vi "Add Application Search Path.vi"(8 "error in":errorcluster, 10 "New Search Path":path) -> (0 "error out":errorcluster, 1 "Added?":bool, 2 "Updated Search Paths":path[](array[path]), 5 "Initial Search Paths":path[](array[path]))   [LabVIEW 2020, in "VI-Hacker.lvlib"]
uses:
  VI-Hacker.lvlib
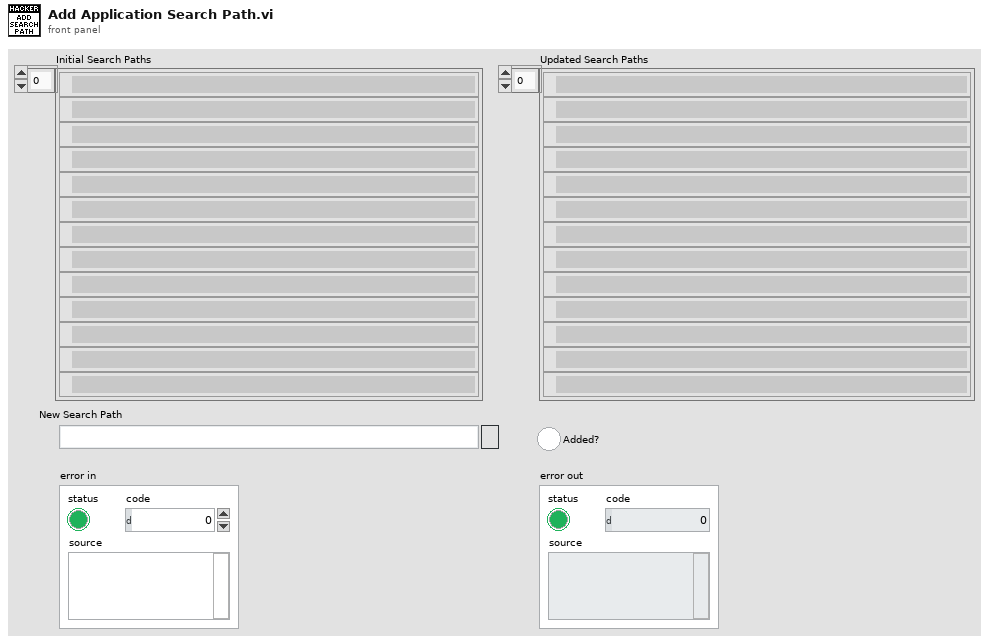
[diagram p1: front panel]
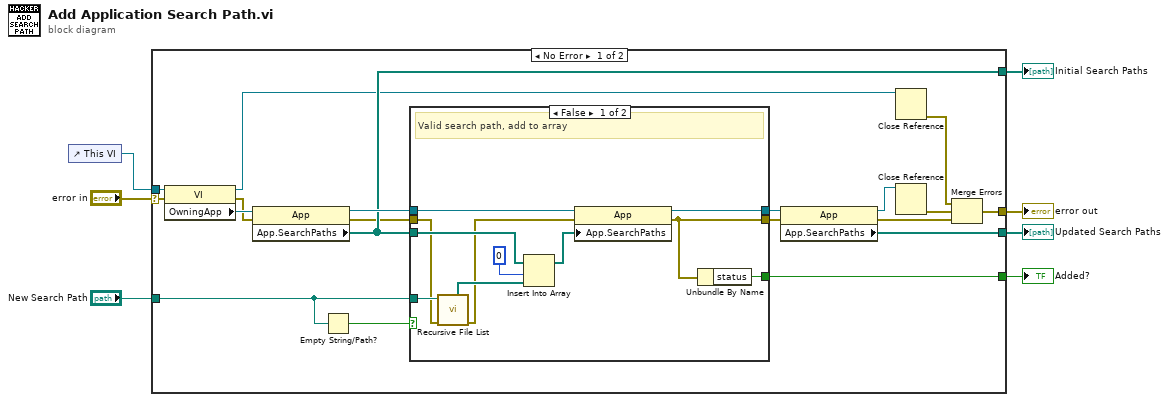
[diagram p0: block diagram]
diagram:
  n1 = control-ref of="This VI"() -> (w7:refnum<vi>)
  n2 = case shown="No Error" "error in" {
    selector: "error in" -> [w19 w40]
    tunnel: w7 -> [w26 _]
    tunnel: [w22 _] -> w6
    tunnel: [w21 _] -> w5
    tunnel: "New Search Path" -> [w8 _]
    tunnel: [w13 w40] -> w2
    tunnel: [w9 _] -> w1
    frame No Error {
      n3 = property class="VI"(reference=w26, error in=w19) -> (reference out=w14:refnum<vi>, error out=w15:errorcluster, "OwningApp"=w25:refnum<vi>)
      n4 = property class="App"(reference=w25, error in=w15) -> (reference out=w24:refnum<vi>, error out=w20:errorcluster, "App.SearchPaths"=w21:path[])
      n5 = Empty String/Path?(string/path=w8) -> (empty?=w10:bool)
      n6 = case shown="False" w10 {
        tunnel: w24 -> [w36 w38]
        tunnel: [w35 w38] -> w23
        tunnel: w21 -> [w34 _]
        tunnel: w20 -> [w28 w39]
        tunnel: w8 -> [w30 _]
        tunnel: [w32 w39] -> w18
        tunnel: [w31 _] -> w9
        frame False {
          # "Valid search path, add to array"
          n7 = call <vilib>:"Recursive File List.vi"("error in (no error)"=w28, "Folder Path"=w30) -> ("error out"=w27:errorcluster, "All Folders"=w29:path[])  [unwired: 5 in, 3 out]
          n8 = Insert Into Array(array=w34, index=0, new element=w29) -> (w37:path[])
          n9 = property class="App"(reference=w36, error in=w27, "App.SearchPaths"=w37) -> (reference out=w35:refnum<vi>, error out=w32:errorcluster)
          n10 = Unbundle By Name(w32) -> ("status"=w31:bool)
        }
        frame True {
          # "New Search Path is invalid"
        }
      }
      n11 = property class="App"(reference=w23, error in=w18) -> (reference out=w16:refnum<vi>, error out=w17:errorcluster, "App.SearchPaths"=w22:path[])
      n12 = Close Reference(reference=w14) -> (error out=w11:errorcluster)  [unwired: 1 in]
      n13 = Close Reference(reference=w16) -> (error out=w12:errorcluster)  [unwired: 1 in]
      n14 = Merge Errors(w11, w12, w17) -> (w13:errorcluster)
    }
    frame Error {
    }
  }
  "Updated Search Paths" <- w6
  "Initial Search Paths" <- w5
  "error out" <- w2
  "Added?" <- w1
